vi "W4 A1.vi"() -> ()   [LabVIEW 2017]
uses:
  Control 1.ctl
panel:
  out "Waveform Chart":dbl(graph)
  in  "Threshold":dbl
  in  "Add to chart Button 2":bool
  in  "Measure Button 2":bool
  out "Measure Value":dbl
  in  "STOP":bool
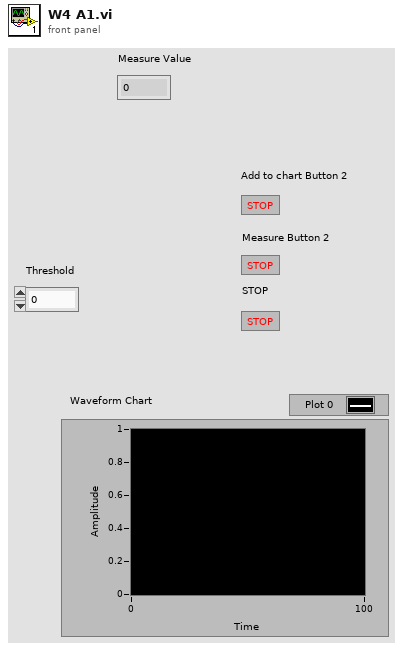
[diagram p1: front panel]
types:
  T1 = typedef "Control 1" = enum16{"Add to chart", "Idle", "Measure"}
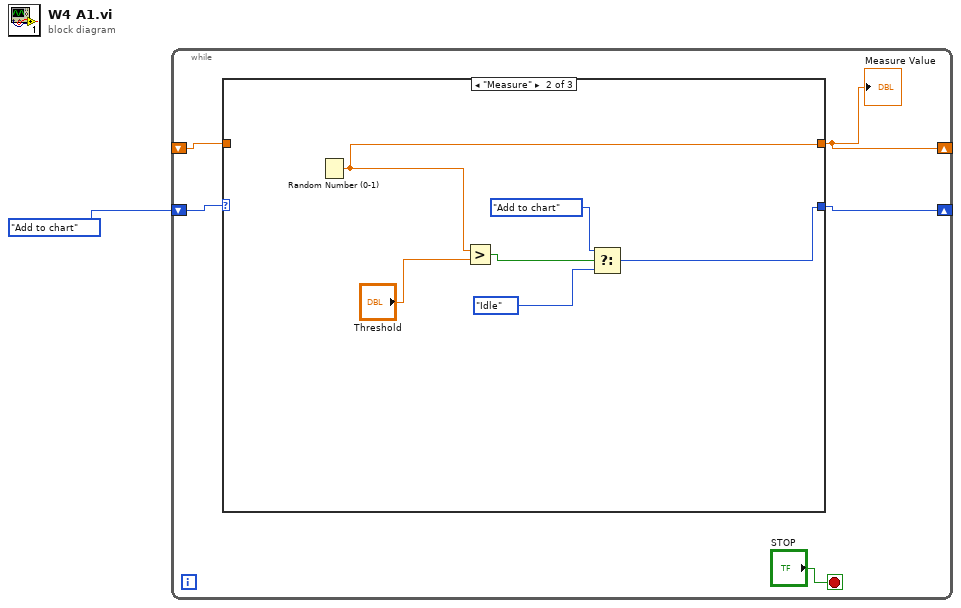
[diagram p0: block diagram]
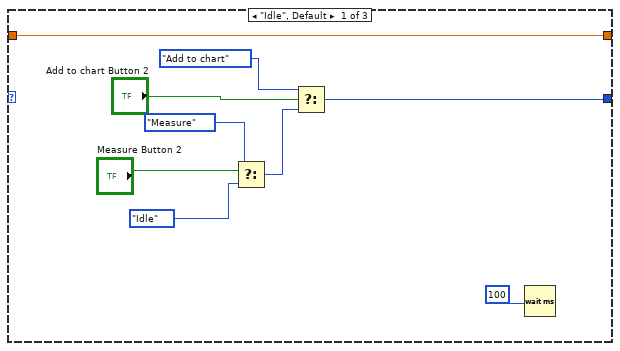
[diagram p2: hidden frame]
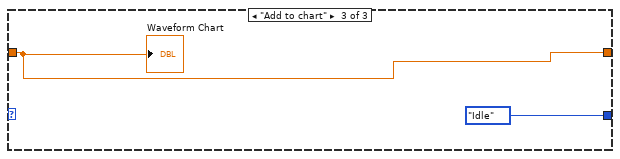
[diagram p3: hidden frame]
diagram:
  n1 = while {
    shift-right: [w2] -> _
    shift-left: Control_1."Add to chart" -> [w6]
    shift-right: [w3] -> _
    shift-left: _ -> [w4]
    stop <- "STOP" stop-if-true
    n2 = case shown="\"Measure\"" w6 {
      tunnel: [w11 w19 Control_1."Idle"] -> w2
      tunnel: w4 -> [w10 _ w22]
      tunnel: [w10 w18 w22] -> w3
      frame "Idle", Default {
        n3 = Select(t=Control_1."Measure", s="Measure Button 2", f=Control_1."Idle") -> (s? t:f=w12:T1)
        n4 = Select(t=Control_1."Add to chart", s="Add to chart Button 2", f=w12) -> (s? t:f=w11:T1)
        n5 = Wait (ms)(milliseconds to wait=100) -> ()  [unwired: 1 out]
      }
      frame "Measure" {
        n6 = Random Number (0-1)() -> (number: 0 to 1=w18:dbl)
        n7 = Greater?(x=w18, y="Threshold") -> (0:w20:bool)
        n8 = Select(t=Control_1."Add to chart", s=w20, f=Control_1."Idle") -> (s? t:f=w19:T1)
      }
      frame "Add to chart" {
        "Waveform Chart" <- w22
      }
    }
    "Measure Value" <- w3
  }
